vi "RC_calibration.vi"(8 "error in (no error)":errorcluster, 11 "VISA resource name":refnum<visa-resource-name>) -> (0 "error IO":errorcluster, 2 "Dynamixel Bounds Out":T1, 3 "VISA resource name out":refnum<visa-resource-name>)   [LabVIEW 2013]
doc: "This code is to set a lower bound on the sail motors and to set the bounds on the rudder motor. You can switch between position control and speed control for the sail motors to cover more distance. The Bound Offset variable determines the travelable range of the motors.\n\nThe VISA resource name should be ASLR3, the Dynamixel USB port.\n\nEric, David, Sean, December 2014"
uses:
  Data/TypeDefs/MotorSetup.ctl
  Data/TypeDefs/DynamixelSetupInfo.ctl
  <instrlib>/Dynamixel Motor/Dynamixel Motor.lvlib
panel:
  in  "Sail 2 Bound Offset":dbl=800.0
  in  "Sail 1 Bound Offset":dbl=800.0
  in  "Stop Calibration":bool
  in  "Dynamixel Bounds Control":T1={"Main Dynamixel Set Data"={"Lower Winch Bound (deg)"=0.0, "Upper Winch Bound (deg)"=0.0}, "Rudder Dynamixel Set Data"={"Lower Winch Bound (deg)"=15.0, "Upper Winch Bound (deg)"=60.0}, "Jib Dynamixel Set Data"={"Lower Winch Bound (deg)"=0.0, "Upper Winch Bound (deg)"=0.0}}
  out "Calibration loop counter":i32
  in  "Sail 2 Calibration Speed":dbl
  in  "Sail 1 Calibration Speed":dbl
  in  "Sail 2 Lower Bound":dbl
  in  "Sail 1 Lower Bound":dbl
  in  "Use Speed\nControl":bool
  out "Position Sail 1":dbl
  out "Position Sail 2":dbl
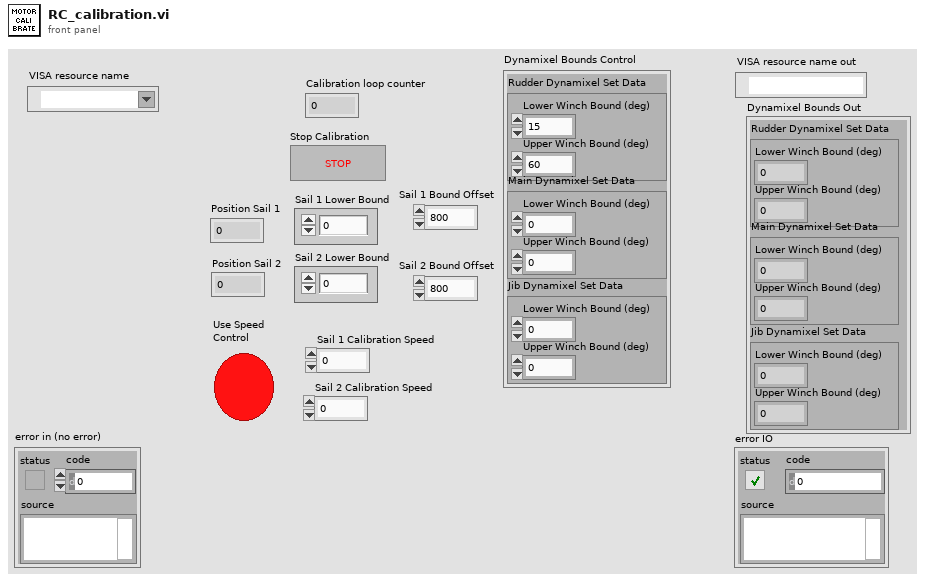
[diagram p1: front panel]
types:
  T1 = typedef "MotorSetup.ctl" = cluster{"Main Dynamixel Set Data":T2, "Rudder Dynamixel Set Data":T2, "Jib Dynamixel Set Data":T2}
  T2 = typedef "DynamixelSetupInfo.ctl" = cluster{"Lower Winch Bound (deg)":dbl, "Upper Winch Bound (deg)":dbl}
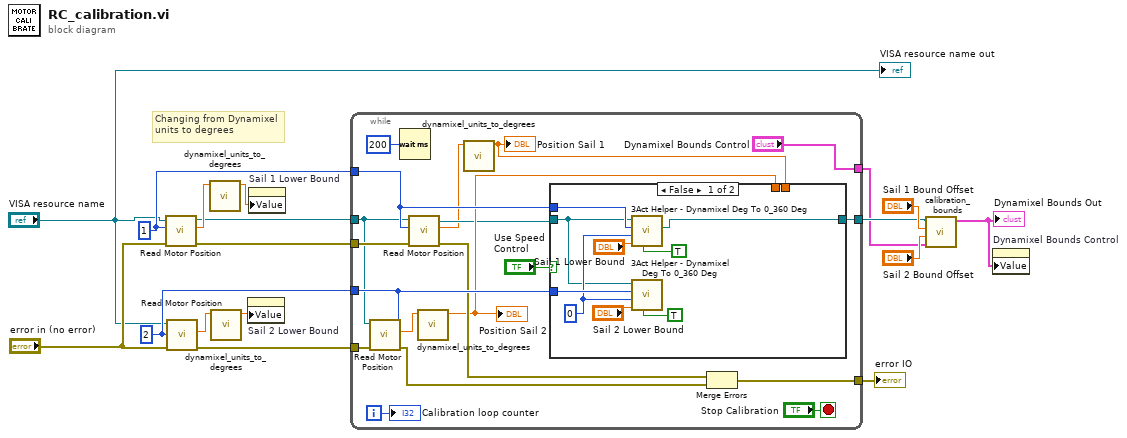
[diagram p0: block diagram]
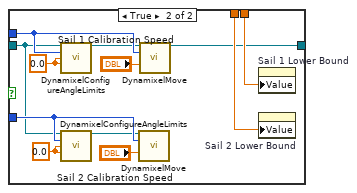
[diagram p2: hidden frame]
diagram:
  w9 = u8 2 ("Motor ID (0)")
  w8 = u8 1 ("Motor ID (0)")
  # "Changing from Dynamixel units to degrees"
  n1 = call <instrlib>:"Read Motor Position.vi"("error in (no error)"="error in (no error)", "Motor ID (0)"=w8, "VISA resource name"="VISA resource name") -> ("error out"=w16:errorcluster, "Position (deg)"=w17:dbl, "VISA resource name out"=w7:refnum<visa-resource-name>)  [unwired: 6 in]
  n2 = call <instrlib>:"Read Motor Position.vi"("error in (no error)"="error in (no error)", "Motor ID (0)"=w9, "VISA resource name"="VISA resource name") -> ("error out"=w15:errorcluster, "Position (deg)"=w12:dbl)  [unwired: 6 in, 1 out]
  n3 = call "dynamixel_units_to_degrees.vi"("Dynamixel Input"=w17) -> ("Degrees"=w14:dbl)  [unwired: 9 in, 1 out]
  n4 = call "dynamixel_units_to_degrees.vi"("Dynamixel Input"=w12) -> ("Degrees"=w13:dbl)  [unwired: 9 in, 1 out]
  n5 = property on="Sail 2 Lower Bound" class="DigNum (strict)"("Value"=w13) -> ()  [unwired: 2 in, 2 out]
  n6 = property on="Sail 1 Lower Bound" class="DigNum (strict)"("Value"=w14) -> ()  [unwired: 2 in, 2 out]
  n7 = while {
    tunnel: w7 -> [w20]
    tunnel: w8 -> [w32]
    tunnel: w9 -> [w31]
    tunnel: ["Dynamixel Bounds Control"] -> w3
    tunnel: w15 -> [w30]
    tunnel: [w27] -> w2
    tunnel: w16 -> [w24]
    tunnel: [w22] -> w4
    i -> [w34]
    stop <- "Stop Calibration" stop-if-true
    n8 = call <instrlib>:"Read Motor Position.vi"("error in (no error)"=w30, "Motor ID (0)"=w31, "VISA resource name"=w20) -> ("error out"=w29:errorcluster, "Position (deg)"=w19:dbl)  [unwired: 6 in, 1 out]
    n9 = Wait (ms)(milliseconds to wait=u32 200) -> ()  [unwired: 1 out]
    n10 = call <instrlib>:"Read Motor Position.vi"("error in (no error)"=w24, "Motor ID (0)"=w32, "VISA resource name"=w20) -> ("error out"=w28:errorcluster, "Position (deg)"=w18:dbl, "VISA resource name out"=w23:refnum<visa-resource-name>)  [unwired: 6 in]
    n11 = call "dynamixel_units_to_degrees.vi"("Dynamixel Input"=w19) -> ("Degrees"=w25:dbl)  [unwired: 9 in, 1 out]
    "Position Sail 2" <- w25
    n12 = call "dynamixel_units_to_degrees.vi"("Dynamixel Input"=w18) -> ("Degrees"=w26:dbl)  [unwired: 9 in, 1 out]
    "Position Sail 1" <- w26
    n13 = case shown="False" "Use Speed\nControl" {
      tunnel: w23 -> [w40 w48]
      tunnel: w32 -> [w45 w50]
      tunnel: w31 -> [w44 w56]
      tunnel: w26 -> [_ w54]
      tunnel: w25 -> [_ w52]
      tunnel: [w39 w46] -> w22
      frame False {
        w41 = 0 ("Dynamixel Cycle Number")
        n14 = call "3Act Helper - Dynamixel Deg To 0_360 Deg.vi"("Motor Read\nCorrectly"=TRUE ("Motor Read\nCorrectly"), "Dynamixel Setpoint In (deg)"="Sail 1 Lower Bound", "Dynamixel Cycle Number"=w41, "Motor ID"=w45, "VISA resource name"=w40) -> ("VISA resource name OUT"=w39:refnum<visa-resource-name>)  [unwired: 4 in, 2 out]
        n15 = call "3Act Helper - Dynamixel Deg To 0_360 Deg.vi"("Motor Read\nCorrectly"=TRUE ("Motor Read\nCorrectly"), "Dynamixel Setpoint In (deg)"="Sail 2 Lower Bound", "Dynamixel Cycle Number"=w41, "Motor ID"=w44, "VISA resource name"=w40) -> ()  [unwired: 4 in, 3 out]
      }
      frame True {
        w51 = 0.0 ("Clockwise Angle Limit (0 deg)")
        w57 = 0.0 ("Clockwise Angle Limit (0 deg)")
        n16 = call "DynamixelConfigureAngleLimits.vi"("VISA resource name"=w48, "Motor ID (0)"=w50, "Clockwise Angle Limit (0 deg)"=w51, "Counter-Clockwise Angle Limit (300 deg)"=w51) -> ("VISA resource name out"=w47:refnum<visa-resource-name>)  [unwired: 10 in, 1 out]
        n17 = call "DynamixelConfigureAngleLimits.vi"("VISA resource name"=w48, "Motor ID (0)"=w56, "Clockwise Angle Limit (0 deg)"=w57, "Counter-Clockwise Angle Limit (300 deg)"=w57) -> ("VISA resource name out"=w53:refnum<visa-resource-name>)  [unwired: 10 in, 1 out]
        n18 = call "DynamixelMove.vi"("VISA resource name"=w53, "Motor ID (0)"=w56, "Goal Speed (RPM)"="Sail 2 Calibration Speed") -> ()  [unwired: 11 in, 2 out]
        n19 = call "DynamixelMove.vi"("VISA resource name"=w47, "Motor ID (0)"=w50, "Goal Speed (RPM)"="Sail 1 Calibration Speed") -> ("VISA resource name out"=w46:refnum<visa-resource-name>)  [unwired: 11 in, 1 out]
        n20 = property on="Sail 1 Lower Bound" class="DigNum (strict)"("Value"=w54) -> ()  [unwired: 2 in, 2 out]
        n21 = property on="Sail 2 Lower Bound" class="DigNum (strict)"("Value"=w52) -> ()  [unwired: 2 in, 2 out]
      }
    }
    n22 = Merge Errors(w28, w29) -> (w27:errorcluster)
    "Calibration loop counter" <- w34
  }
  "error IO" <- w2
  n23 = call "calibration_bounds.vi"("Dynamixel Bounds"=w3, "Sail 2 Bound Offset"="Sail 2 Bound Offset", "Sail 1 Bound Offset"="Sail 1 Bound Offset", "VISA resource name in"=w4) -> ("Dynamixel Bounds Out"=w1:T1)  [unwired: 7 in]
  "Dynamixel Bounds Out" <- w1
  n24 = property on="Dynamixel Bounds Control" class="Clust (strict)"("Value"=w1) -> ()  [unwired: 2 in, 2 out]
  "VISA resource name out" <- "VISA resource name"
